vi "_Update Graph.vi"(4 "TIC (F)":bool, 5 "Auto Scale":bool, 6 "Graph Ref":refnum<vi>, 7 "Data":T2, 8 "error in (no error)":errorcluster, 9 "Log Scale":bool, 10 "CPS":bool, 11 "Averaging":bool) -> (3 "Graph Property":T1)   [LabVIEW 2012]
uses:
  Type/_Data.ctl
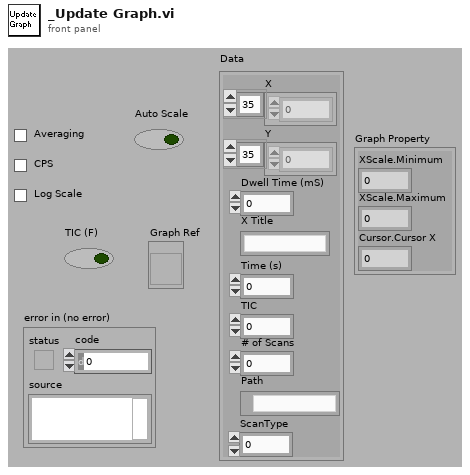
[diagram p1: front panel]
types:
  T1 = cluster{"XScale.Minimum":dbl, "XScale.Maximum":dbl, "Cursor.Cursor X":dbl}
  T2 = typedef "_Data.ctl" = cluster{"X":dbl[], "Y":dbl[], "Dwell Time (mS)":dbl, "X Title":string, "Time (s)":dbl, "TIC":u32, "# of Scans":i32, "Path":path, "ScanType":i32}
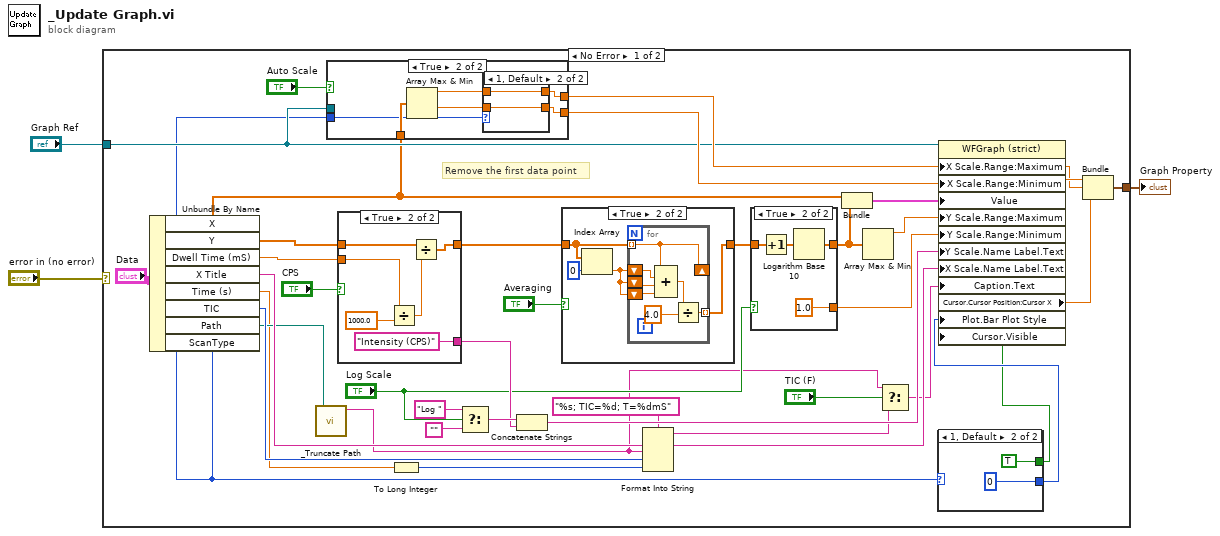
[diagram p0: block diagram]
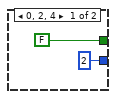
[diagram p2: hidden frame]
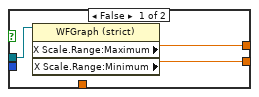
[diagram p3: hidden frame]
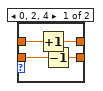
[diagram p4: hidden frame]
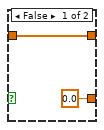
[diagram p5: hidden frame]
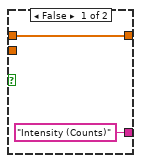
[diagram p7: hidden frame]
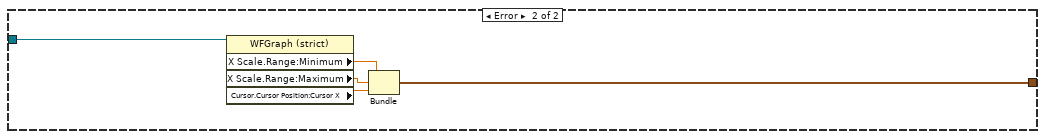
[diagram p8: hidden frame]
diagram:
  n1 = case shown="No Error" "error in (no error)" {
    tunnel: [w19 w87] -> w1
    tunnel: "Graph Ref" -> [w16 w90]
    frame No Error {
      # "Remove the first data point"
      n2 = Unbundle By Name("Data") -> ("X"=w12:dbl[], "Y"=w9:dbl[], "Dwell Time (mS)"=w30:dbl, "X Title"=w27:string, "Time (s)"=w15:dbl, "TIC"=w26:u32, "Path"=w24:path, "ScanType"=w10:i32)
      n3 = call "_Truncate Path.vi"("Path"=w24) -> ("String"=w4:string)  [unwired: 1 in, 5 out]
      n4 = case shown="True" "Auto Scale" {
        tunnel: w12 -> [_ w53]
        tunnel: [w46 w48] -> w23
        tunnel: [w47 w49] -> w22
        tunnel: w16 -> [w45 _]
        tunnel: w10 -> [_ w52]
        frame False {
          n5 = property class="WFGraph (strict)"(reference=w45) -> ("X Scale.Range:Maximum"=w47:dbl, "X Scale.Range:Minimum"=w46:dbl)  [unwired: 1 in, 2 out]
        }
        frame True {
          n6 = Array Max & Min(array=w53) -> (max value=w51:dbl, min value=w50:dbl)  [unwired: 2 out]
          n7 = case shown="1, Default" w52 {
            tunnel: w51 -> [w57 w59]
            tunnel: w50 -> [w55 w58]
            tunnel: [w56 w59] -> w49
            tunnel: [w54 w58] -> w48
            frame 0, 2, 4 {
              n8 = Increment(x=w57) -> (x+1=w56:dbl)
              n9 = Decrement(x=w55) -> (x-1=w54:dbl)
            }
            frame 1, Default {
            }
          }
        }
      }
      n10 = case shown="True" "CPS" {
        tunnel: w9 -> [w79 w84]
        tunnel: [w79 w82] -> w13
        tunnel: ["Intensity (Counts)" "Intensity (CPS)"] -> w35
        tunnel: w30 -> [_ w80]
        frame False {
        }
        frame True {
          n11 = Divide(x=w80, y=1000.0) -> (x/y=w83:dbl)
          n12 = Divide(x=w84, y=w83) -> (x/y=w82:dbl[])
        }
      }
      n13 = To Long Integer(number=w15) -> (32bit integer=w14:i32)
      n14 = Select(t="Log ", s="Log Scale", f="") -> (s? t:f=w36:string)
      n15 = Concatenate Strings(w36, w35) -> (w28:string)
      n16 = case shown="True" "Averaging" {
        tunnel: w13 -> [w66 w68]
        tunnel: [w66 w67] -> w34
        frame False {
        }
        frame True {
          n17 = Index Array(array=w68, index=0) -> (element=w69:dbl)
          n18 = for {
            shift-right: [w74] -> _
            shift-left: w69 -> [w77]
            shift-left: w69 -> [w76]
            shift-left: w69 -> [w75]
            tunnel: w68 -> [w74] mode=indexing
            tunnel: [w71] -> w67 mode=indexing
            n19 = Compound Arithmetic op=ADD(w74, w77, w76, w75) -> (w73:dbl)
            n20 = Divide(x=w73, y=4.0) -> (x/y=w71:dbl)
          }
        }
      }
      n21 = Format Into String(format string="%s; TIC=%d; T=%dmS", w4, w26, w14) -> (resulting string=w6:string)  [unwired: 2 in, 1 out]
      n22 = case shown="True" "Log Scale" {
        tunnel: w34 -> [w61 w65]
        tunnel: [w61 w64] -> w33
        tunnel: [0.0 ("y") 1.0 ("y")] -> w21
        frame False {
        }
        frame True {
          n23 = Increment(x=w65) -> (x+1=w62:dbl[])
          n24 = Logarithm Base 10(1:w62) -> (0:w64:dbl[])
        }
      }
      n25 = Bundle("X"=w12, "Y"=w33) -> (w29:cluster{"X":dbl[], "Y":dbl[]})  [unwired: 1 out]
      n26 = Array Max & Min(array=w33) -> (max value=w20:dbl)  [unwired: 3 out]
      n27 = Select(t=w4, s="TIC (F)", f=w6) -> (s? t:f=w5:string)
      n28 = case shown="1, Default" w10 {
        tunnel: [u8 2 ("Plot.Bar Plot Style") u8 0 ("Plot.Bar Plot Style")] -> w11
        tunnel: [FALSE TRUE] -> w8
        frame 0, 2, 4 {
        }
        frame 1, Default {
        }
      }
      n29 = property class="WFGraph (strict)"(reference=w16, "X Scale.Range:Maximum"=w22, "X Scale.Range:Minimum"=w23, "Value"=w29, "Y Scale.Range:Maximum"=w20, "Y Scale.Range:Minimum"=w21, "Y Scale.Name Label.Text"=w28, "X Scale.Name Label.Text"=w27, "Caption.Text"=w5, "Plot.Bar Plot Style"=w11, "Cursor.Visible"=w8) -> ("Cursor.Cursor Position:Cursor X"=w18:dbl)  [unwired: 1 in, 2 out]
      n30 = Bundle("XScale.Minimum"=w23, "XScale.Maximum"=w22, "Cursor.Cursor X"=w18) -> (w19:T1)  [unwired: 1 out]
    }
    frame Error {
      n31 = property class="WFGraph (strict)"(reference=w90) -> ("X Scale.Range:Minimum"=w89:dbl, "X Scale.Range:Maximum"=w88:dbl, "Cursor.Cursor Position:Cursor X"=w86:dbl)  [unwired: 1 in, 2 out]
      n32 = Bundle("XScale.Minimum"=w89, "XScale.Maximum"=w88, "Cursor.Cursor X"=w86) -> (w87:T1)  [unwired: 1 out]
    }
  }
  "Graph Property" <- w1
